vi "OCR.vi"(7 "error in":errorcluster) -> (27 "error out":errorcluster)   [LabVIEW 2018]
uses:
  <vilib>/userdefined/High Color/IMAQdx.ctl
  <vilib>/vision/OCR.llb/IMAQ OCR Session.ctl
  <vilib>/vision/NI_Vision_Development_Module.lvlib
  <vilib>/vision/driver/NI_Vision_Acquisition_Software.lvlib
panel:
  in  "정지 버튼":bool
  out "Read String":string
  out "IMAQ OCR Session (dup)":T1
  in  "Session In":T2
  out "Image Out":T3(plugin-control)
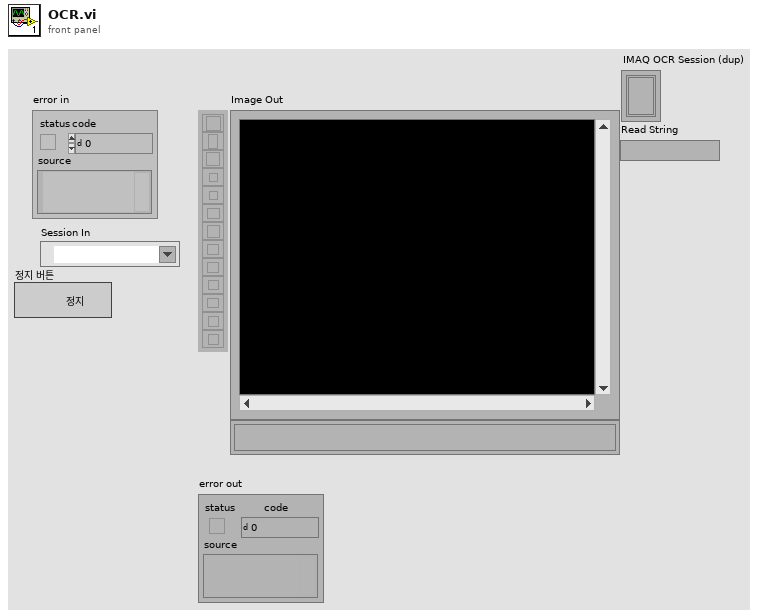
[diagram p1: front panel]
types:
  T1 = typedef "IMAQ OCR Session.ctl" = refnum<k1>
  T2 = typedef "IMAQdx.ctl" = refnum<k21>
  T3 = typedef "IMAQ Image.ctl" = refnum<image>
  T4 = cluster{"Threshold Data":cluster{"Method":enum16{"Fixed Range", "Uniform", "Linear", "Non Linear", "Local", "Color"}, "Looking for":u32, "Color Mode":u32, "Kernel Size":cluster{"Width":i32, "Height":i32}, "Ranges":cluster{"Min":i32, "Max":i32}[]}, "Reject Border":bool, "Number Of Erosions":i32, "Size & Spacing":cluster{"Segment Algorithm":u16, "Min Bounding Rect Width":i32, "Max Bounding Rect Width":i32, "Min Bounding Rect Height":i32, "Max Bounding Rect Height":i32, "Min Character Size":i32, "Max Character Size":i32, "Min Char Spacing":i32, "Max Horiz Element Spacing":i32, "Max Vert Element Spacing":i32, "Max Space Distance":i32}, "Read Options":cluster{"Read Strategy":i32, "Read Resolution":i32, "Scale Dependant":bool, "Aspect Ratio":i32, "Acceptance Level":i32, "Substitution Character":string, "MultiLine":bool}, "Valid Characters":cluster{"Pre-defined characters":i32, "User-defined characters":string}[], "Use Text Pattern":bool, "Orientation":u32, "# Lines Expected":u32, "Number of Blocks":i32}
  T5 = typedef "Image Type" = u32
  T6 = cluster{"Global Rectangle":i32[], "Contours":cluster{"Contour Type":u32, "ROI Type":u32, "Points":i32[]}[]}
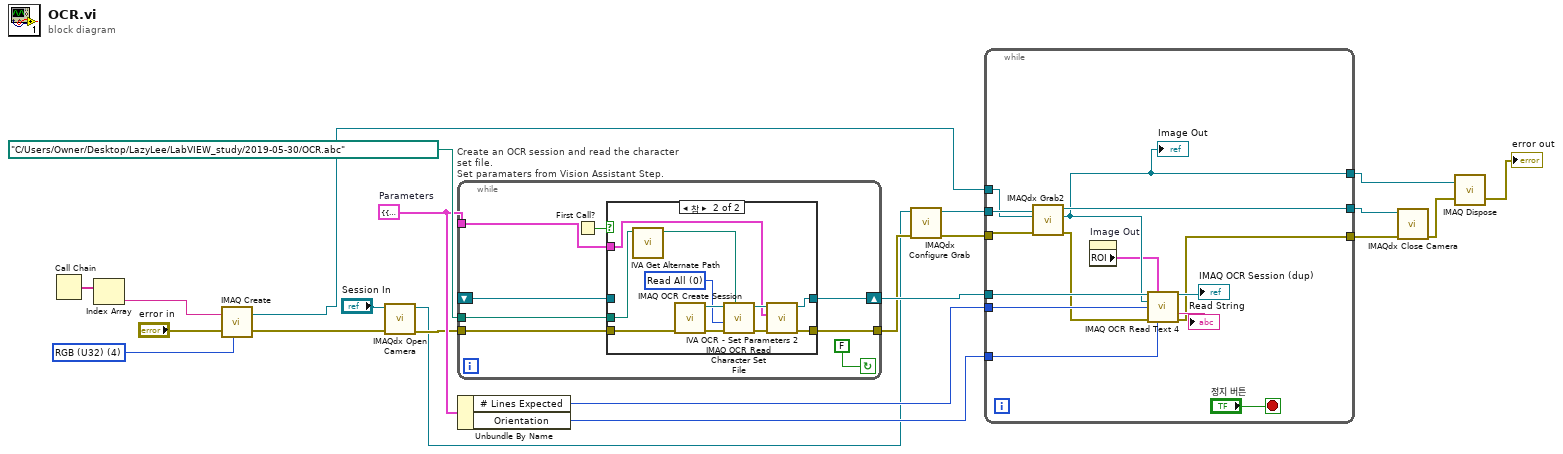
[diagram p0: block diagram]
diagram:
  w17 = T4 {"Threshold Data"={"Method"=enum."Uniform", "Looking for"=1, "Color Mode"=0, "Kernel Size"={"Width"=32, "Height"=32}, "Ranges"=[{"Min"=1, "Max"=255}]}, "Reject Border"=TRUE, "Number Of Erosions"=0, "Size & Spacing"={"Segment Algorithm"=0, "Min Bounding Rect Width"=1, "Max Bounding Rect Width"=65536, "Min Bounding Rect Height"=1, "Max Bounding Rect Height"=65536, "Min Character Size"=20, "Max Character Size"=65536, "Min Char Spacing"=1, "Max Horiz Element Spacing"=1, "Max Vert Element Spacing"=0, "Max Space Distance"=65536}, "Read Options"={"Read Strategy"=1, "Read Resolution"=2, "Scale Dependant"=FALSE, "Aspect Ratio"=400, "Acceptance Level"=700, "Substitution Character"="?", "MultiLine"=TRUE}, "Valid Characters"=[], "Use Text Pattern"=FALSE, "Orientation"=0, "# Lines Expected"=0, "Number of Blocks"=4}  # Parameters
  w19 = T5 4 items=["Grayscale (U8)", "Grayscale (I16)", "Grayscale (SGL)", "Complex (CSG)", "RGB (U32)", "HSL (U32)", "RGB (U64)", "Grayscale (U16)"] ("Image Type")
  n1 = Call Chain() -> (call chain=w21:string[])
  n2 = Index Array(array=w21) -> (element=w20:string)  [unwired: 1 in]
  n3 = call "IMAQ Create"("Image Name"=w20, "Image Type"=w19, "error in (no error)"="error in") -> ("New Image"=w2:T3, "error out"=w1:errorcluster)  [unwired: 1 in, 1 out]
  n4 = call <vilib>:"IMAQdx Open Camera.vi"("error in"=w1, "Session In"="Session In") -> ("error out"=w10:errorcluster, "Session Out"=w9:T2)  [unwired: 8 in]
  n5 = while "Create an OCR session and read the character set file.\nSet paramaters from Vision Assistant Step." {
    shift-right: [w27] -> w16
    shift-left: _ -> [w26]
    tunnel: w10 -> [w29]
    tunnel: w17 -> [w25]
    tunnel: path "C:/Users/Owner/Desktop/LazyLee/LabVIEW_study/2019-05-30/OCR.abc" ("File Path") -> [w24]
    tunnel: [w23] -> w12
    stop <- FALSE continue-if-true
    n6 = First Call?() -> (First Call?: T/F=w28:bool)
    n7 = case "케이스 구조" shown="참" w28 {
      tunnel: w24 -> [_ w36]
      tunnel: w29 -> [w31 w40]
      tunnel: [w32 w38] -> w27
      tunnel: [w31 w37] -> w23
      tunnel: w25 -> [_ w33]
      tunnel: w26 -> [w32 _]
      frame False {
      }
      frame True {
        w41 = 0 items=["Read All", "Read Character Set Only", "Read Properties Only"] ("Read Options")
        n8 = call <vilib>:"IVA Get Alternate Path.vi"("Path In"=w36) -> ("Path Out"=w35:path)  [unwired: 10 out]
        n9 = call "IMAQ OCR Create Session"("error in (no error)"=w40) -> ("error out"=w42:errorcluster, "IMAQ OCR Session"=w43:T1)  [unwired: 9 out]
        n10 = call "IMAQ OCR Read Character Set File"("File Path"=w35, "error in (no error)"=w42, "Read Options"=w41, "IMAQ OCR Session"=w43) -> ("error out"=w39:errorcluster, "IMAQ OCR Session (dup)"=w34:T1)  [unwired: 1 in, 5 out]
        n11 = call <vilib>:"IVA OCR - Set Parameters 2.vi"("error in (no error)"=w39, "Parameters"=w33, "IMAQ OCR Session"=w34) -> ("error out"=w37:errorcluster, "IMAQ OCR Session Out"=w38:T1)  [unwired: 7 in]
      }
    }
  }
  n12 = Unbundle By Name(w17) -> ("# Lines Expected"=w14:u32, "Orientation"=w15:u32)
  n13 = call <vilib>:"IMAQdx Configure Grab.vi"("error in"=w12, "Session In"=w9) -> ("error out"=w11:errorcluster, "Session Out"=w8:T2)  [unwired: 8 in]
  n14 = while {
    tunnel: w16 -> [w57]
    tunnel: w15 -> [w56]
    tunnel: w14 -> [w55]
    tunnel: w2 -> [w46]
    tunnel: w11 -> [w53]
    tunnel: w8 -> [w54]
    tunnel: [w49] -> w7
    tunnel: [w45] -> w4
    tunnel: [w47] -> w6
    stop <- "정지 버튼" stop-if-true
    n15 = call <vilib>:"IMAQdx Grab2.vi"("error in"=w53, "Image In"=w46, "Session In"=w54) -> ("error out"=w52:errorcluster, "Image Out"=w45:T3, "Session Out"=w49:T2)  [unwired: 5 in, 1 out]
    "Image Out" <- w45
    n16 = property on="Image Out" class="ImageControl"() -> ("ROI"=w44:T6)  [unwired: 2 in, 2 out]
    n17 = call "IMAQ OCR Read Text 4"("IMAQ OCR Session"=w57, "ROI Descriptor"=w44, "Image"=w45, "Number of Lines Requested"=w55, "error in (no error)"=w52, "Orientation"=w56) -> ("IMAQ OCR Session (dup)"=→"IMAQ OCR Session (dup)":T1, "Read String"=→"Read String":string, "error out"=w47:errorcluster)  [unwired: 7 out]
  }
  n18 = call <vilib>:"IMAQdx Close Camera.vi"("error in"=w6, "Session In"=w7) -> ("error out"=w5:errorcluster)  [unwired: 9 in]
  n19 = call "IMAQ Dispose"("Image"=w4, "error in (no error)"=w5) -> ("error out"=→"error out":errorcluster)  [unwired: 4 in]
